vi "Waveform, Remove Noise.vi"(0 "error in":errorcluster, 1 "lower limit (-0.05)":dbl=-0.05, 2 "upper limit (0.05)":dbl=0.05, 3 "waveform":waveform(dbl)={"t0"=timestamp(3476124967.3590007 s since 1904-01-01), "dt"=5e-07, "Y"=[], "attributes"=variant("Average Size"=variant(dbl 30.0), "Frequency (Hz)"=variant(dbl 934.2869670050022), "Interphase Delay (us)"=variant(dbl 9544.155), "Number of Samples"=variant(dbl 320000.0), "Process Timestamp"=variant(dbl 3476124968.578125), "Recvy Amp (V)"=variant(dbl 1.4945756092317695), "Recvy Amp (mA)"=variant(dbl 2.9939666785417054), "Recvy Duty Factor"=variant(dbl 0.07497960063993174), "Recvy Frequency (Hz)"=variant(dbl 50.005863474295865), "Recvy Period (us)"=variant(dbl 19997.654885292053), "Recvy Pulse Width (us)"=variant(dbl 1499.416177034378), "Recvy Trigger (s)"=variant(dbl 0.017093499999999998), "Resistance (ohms)"=variant(dbl 499.195806), "Sample Frequency (MHz)"=variant(dbl 2.0), "Stim Amp (V)"=variant(dbl -7.721513463541287e-05), "Stim Amp (mA)"=variant(dbl -0.00015467905320385017), "Stim Duty Factor"=variant(dbl 0.00667870665716196), "Stim Frequency (Hz)"=variant(dbl 1818.5680705357086), "Stim Period (us)"=variant(dbl 549.8831834793091), "Stim Pulse Width (us)"=variant(dbl 3.672508478164673), "Stim Trigger (s)"=variant(dbl 0.0068975), "dt (us)"=variant(dbl 0.5))}) -> (7 "error out":errorcluster, 10 "waveform out":waveform(dbl)={"t0"=timestamp(0 s since 1904-01-01), "dt"=nan, "Y"=[]})   [LabVIEW 2010]
doc: "This function removes any data (noise) in a waveform that is within the upper and lower limits."
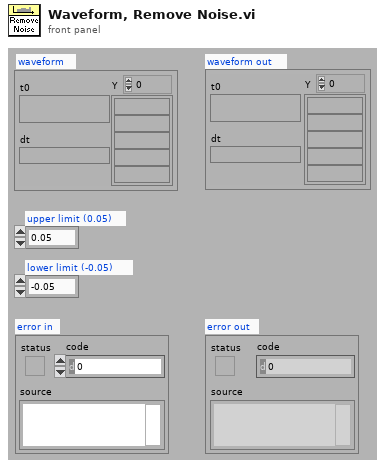
[diagram p1: front panel]
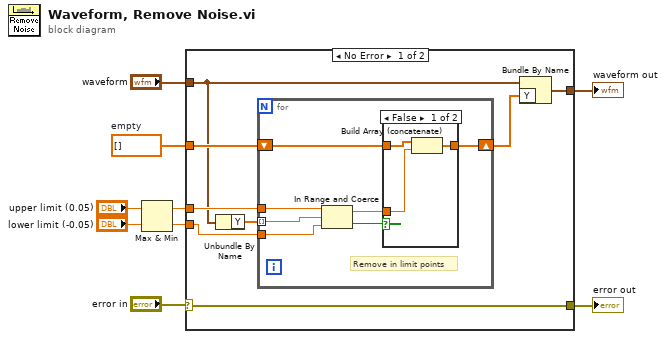
[diagram p0: block diagram]
diagram:
  w9 = dbl[] []  # empty
  n1 = Max & Min(x="upper limit (0.05)", y="lower limit (-0.05)") -> (max(x,y)=w2:dbl, min(x,y)=w1:dbl)
  n2 = case shown="No Error" "error in" {
    selector: "error in" -> [w11 w30]
    tunnel: w2 -> [w16 _]
    tunnel: w9 -> [w15 _]
    tunnel: "waveform" -> [w13 w29]
    tunnel: [w12 w29] -> w5
    tunnel: [w11 w30] -> w6
    tunnel: w1 -> [w10 _]
    frame No Error {
      n3 = Unbundle By Name(w13) -> ("Y"=w17:dbl[])
      n4 = for {
        tunnel: w17 -> [w21] mode=indexing
        tunnel: w10 -> [w20]
        tunnel: w16 -> [w22]
        shift-right: [w24] -> w14
        shift-left: w15 -> [w23]
        # "Remove in limit points"
        n5 = In Range and Coerce(upper limit=w22, x=w21, lower limit=w20) -> (coerced(x)=w18:dbl, In Range?=w19:bool)
        n6 = case shown="False" w19 {
          tunnel: [w27 w28] -> w24
          tunnel: w23 -> [w26 w28]
          tunnel: w18 -> [w25 _]
          frame False {
            n7 = Build Array (concatenate)(w26, w25) -> (w27:dbl[])
          }
          frame True {
          }
        }
      }
      n8 = Bundle By Name(cluster=w13, "Y"=w14) -> (w12:waveform(dbl))
    }
    frame Error {
    }
  }
  "waveform out" <- w5
  "error out" <- w6
